vi "SQLNumResultCols.vi"(4 "error in (no error)":errorcluster, 7 "InputHandle":i32) -> (0 "error out":errorcluster, 2 "NumResultCols":i32, 3 "OutputHandle":i32)   [LabVIEW 2011]
doc: "Donne le nombre de colonnes résultant de l'exécution de la requête"
uses:
  Odbc32.dll
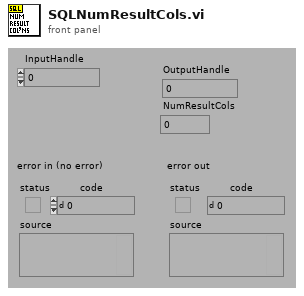
[diagram p1: front panel]
types:
  T1 = enum16{"NOPE", "SQL_HANDLE_ENV", "SQL_HANDLE_DBC", "SQL_HANDLE_STMT", "SQL_HANDLE_DESC"}
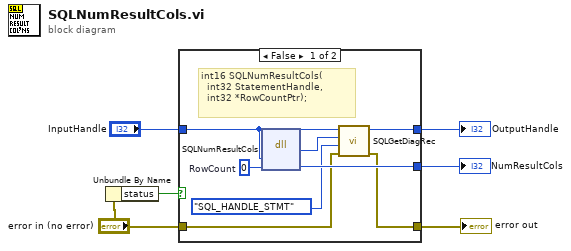
[diagram p0: block diagram]
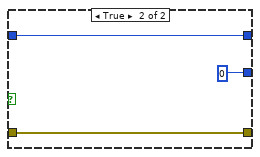
[diagram p2: hidden frame]
diagram:
  n1 = Unbundle By Name("error in (no error)") -> ("status"=w2:bool)
  n2 = case shown="False" w2 {
    tunnel: [w13 0] -> w6
    tunnel: "InputHandle" -> [w11 w15]
    tunnel: [w10 w15] -> w4
    tunnel: [w8 w17] -> w1
    tunnel: "error in (no error)" -> [w9 w17]
    frame False {
      w14 = 0  # RowCount
      # "int16 SQLNumResultCols(\n  int32 StatementHandle, \n  int32 *RowCountPtr);"
      n3 = dll-call lib="Odbc32.dll" fn="SQLNumResultCols"("StatementHandle"=w11, "RowCountPtr"=w14) -> (w12:i16, "RowCountPtr"=w13:i32)  [unwired: 4 in, 2 out]
      n4 = call "SQLGetDiagRec.vi"("error in (no error)"=w9, "HandleType"=T1."SQL_HANDLE_STMT", "Status (SQL_SUCCESS=0)"=w12, "Input Handle"=w11) -> ("error out"=w8:errorcluster, "Output Handle"=w10:i32)  [unwired: 2 out]
    }
    frame True {
    }
  }
  "NumResultCols" <- w6
  "OutputHandle" <- w4
  "error out" <- w1
